vi "elab pictures 2d.vi"(8 "error in":errorcluster, 11 "path file in":path) -> (0 "error out":errorcluster)   [LabVIEW 2023]
uses:
  listbox/Selection Global Method.ctl
  <vilib>/Utility/file.llb/Read Delimited Spreadsheet (I64).vi
  queue/Front Panel Message Queue.lvlib
panel:
  in  "generate":bool
  in  "reset":bool
  out "all rows 2":i32[][][](array[numeric])
  out "all rows":i32[][][](array[numeric])
  in  "List Selected":T1(array[cluster])
  out "List Selected v":string[](array[string])
  out "List File":i32(listbox)
  in  "load":bool
  in  "Stop":bool
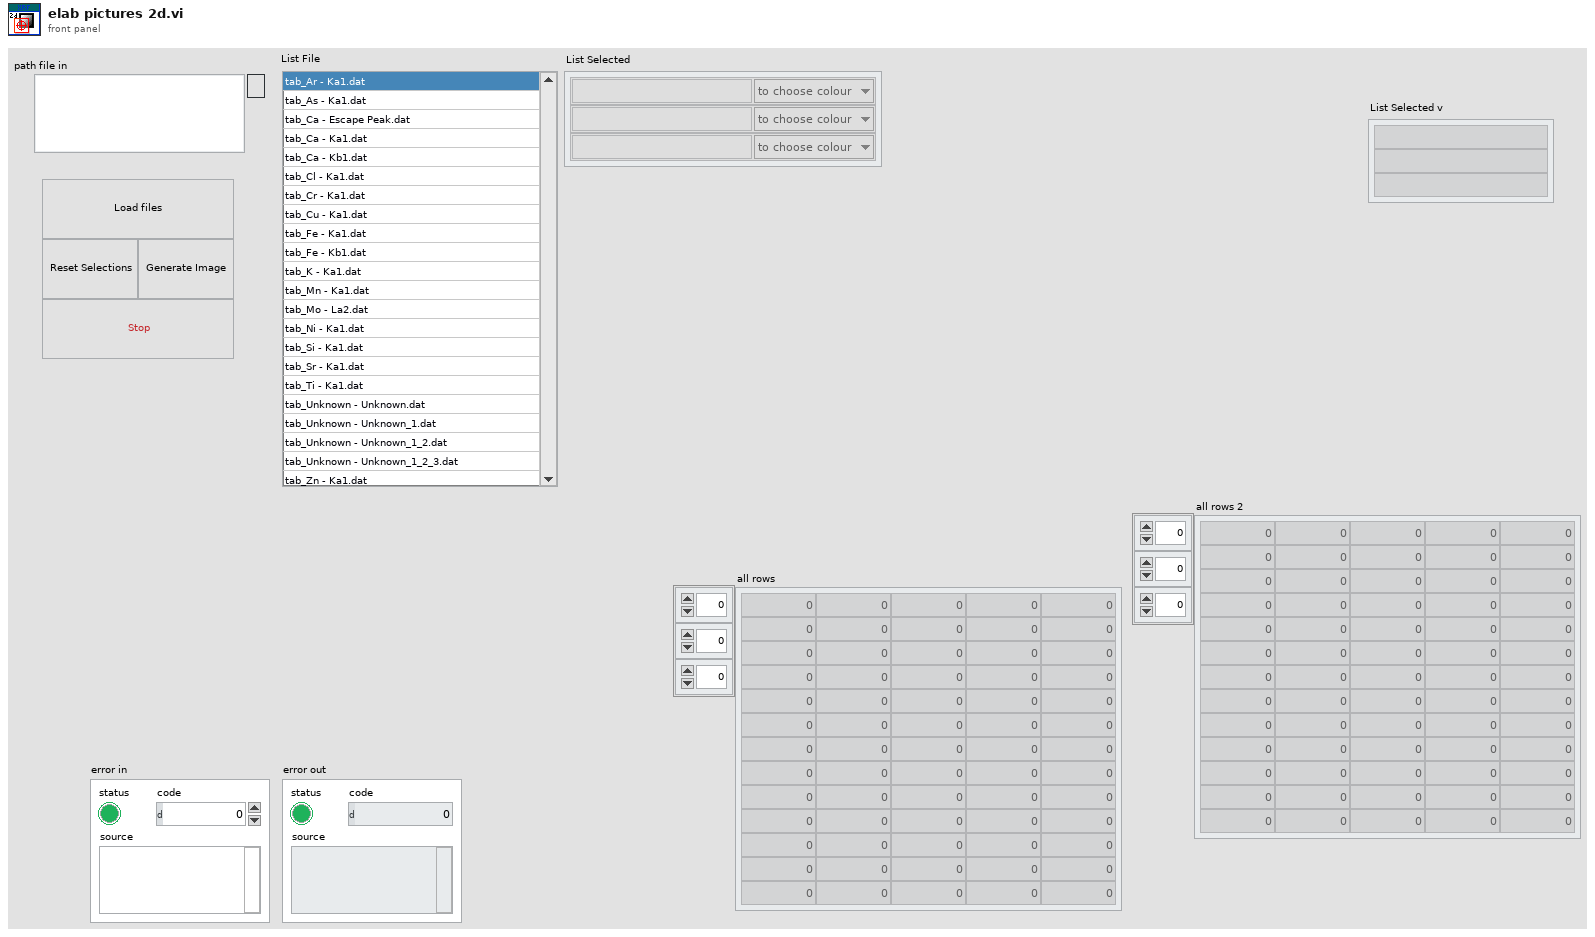
[diagram p1: front panel]
types:
  T1 = cluster{"Table":string, "color":enum16{"to choose colour", "red", "green", "blue"}}[]
  T2 = typedef "Front Panel Message Queue.lvlib/2d3d Message Queues.ctl" = cluster{"Main":refnum<queue>, "2d":refnum<queue>, "3d":refnum<queue>}
  T3 = typedef "Selection Global Method.ctl" = enum16{"Read Selection", "Force Selection", "Mouse Down Event", "Select All", "Select None", "Invert Selection", "Read Selection and Tags"}
  T4 = cluster{"Red name":string, "Green name":string, "Blu name":string}
  T5 = cluster{"Table":string, "color":enum16{"to choose colour", "red", "green", "blue"}}
  T6 = enum16{"to choose colour", "red", "green", "blue"}
  T7 = typedef "LVPoint32TypeDef.ctl" = cluster{"Horizontal":i32, "Vertical":i32}
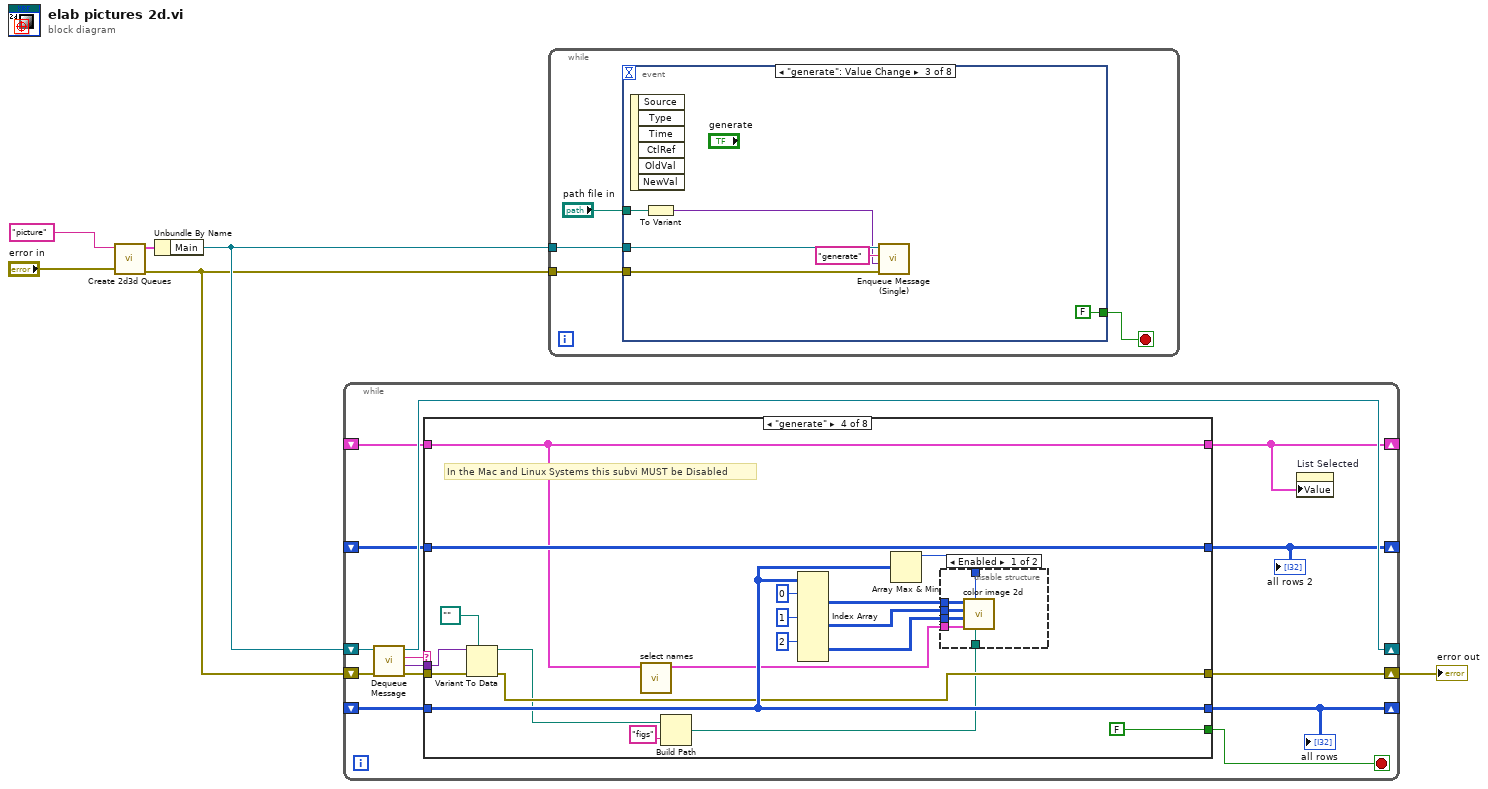
[diagram p0: block diagram]
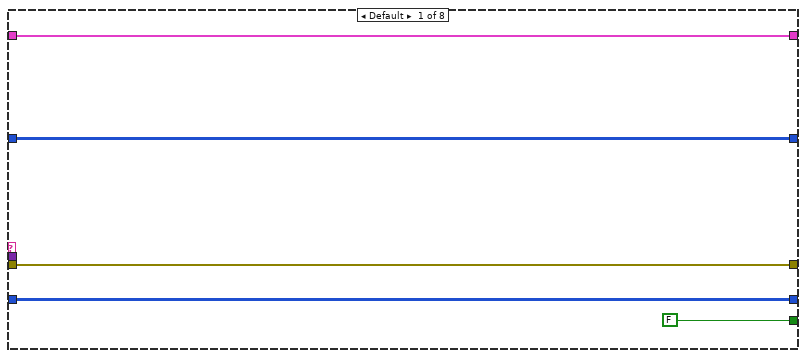
[diagram p2: hidden frame]
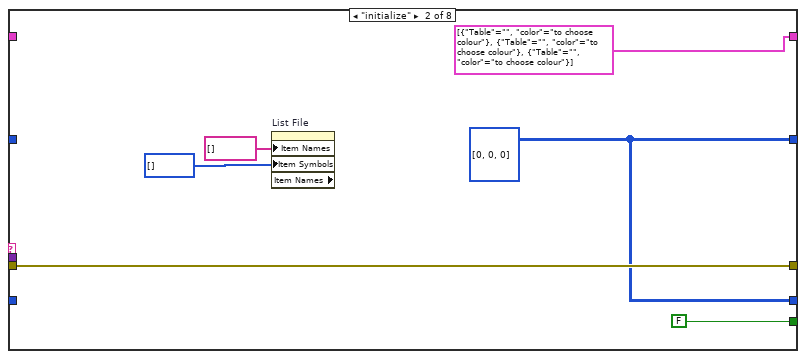
[diagram p3: hidden frame]
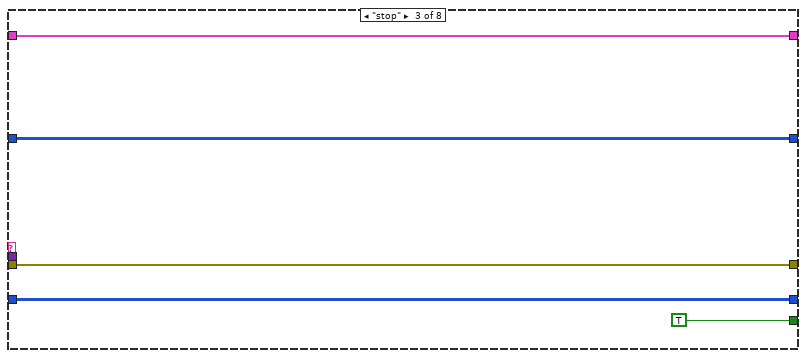
[diagram p4: hidden frame]
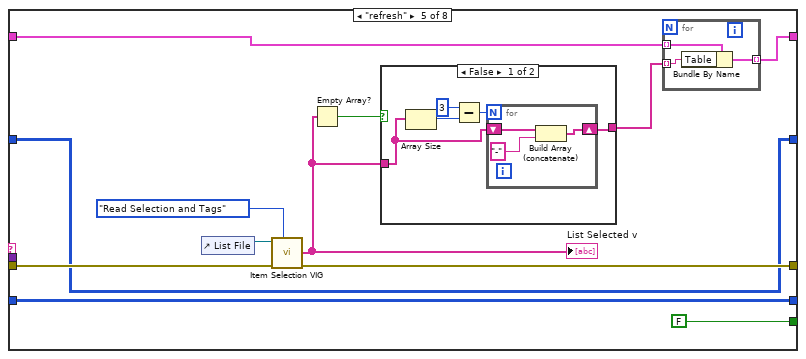
[diagram p6: hidden frame]
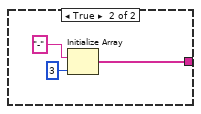
[diagram p7: hidden frame]
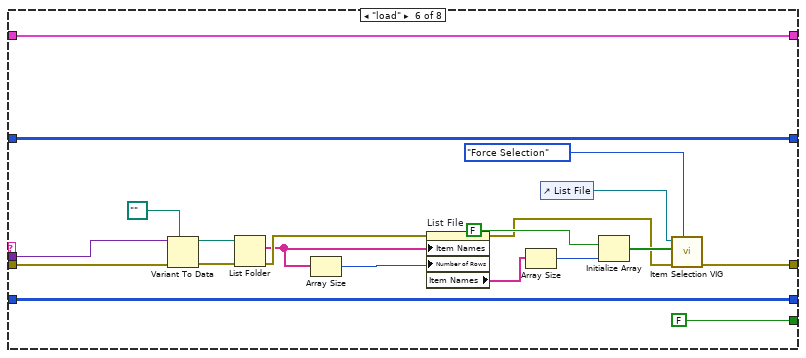
[diagram p8: hidden frame]
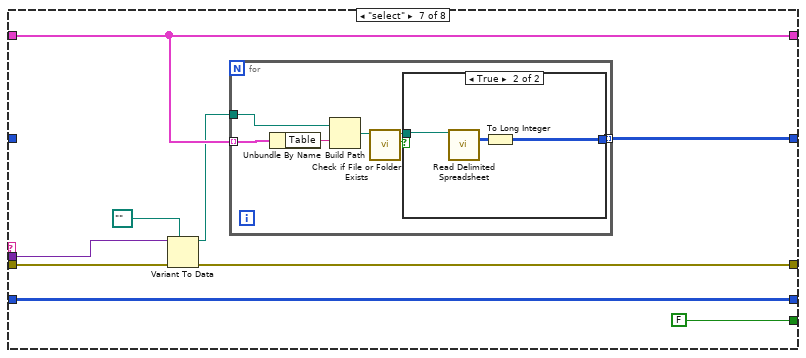
[diagram p9: hidden frame]
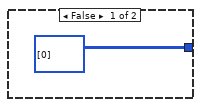
[diagram p10: hidden frame]
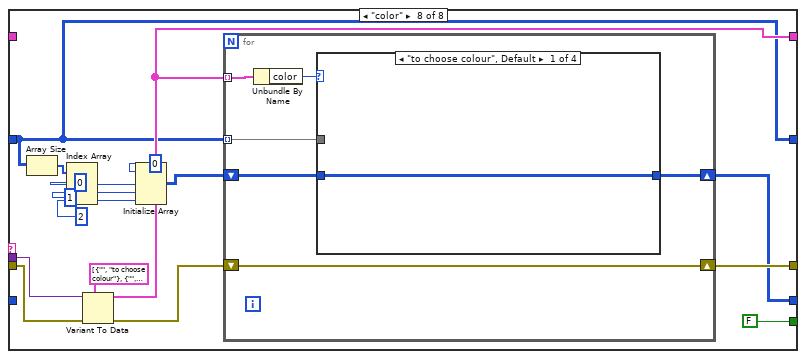
[diagram p11: hidden frame]
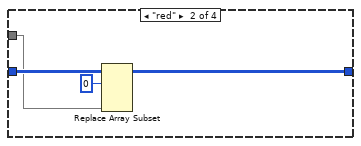
[diagram p12: hidden frame]
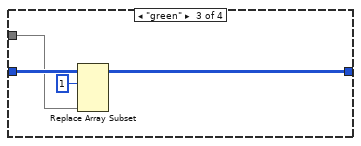
[diagram p13: hidden frame]
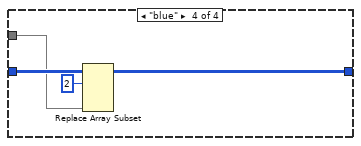
[diagram p14: hidden frame]
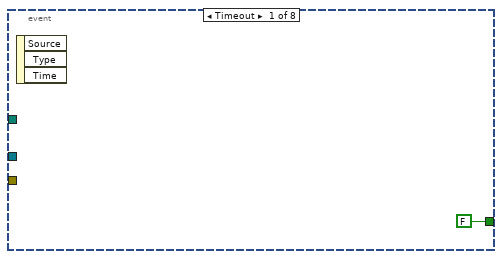
[diagram p15: hidden frame]
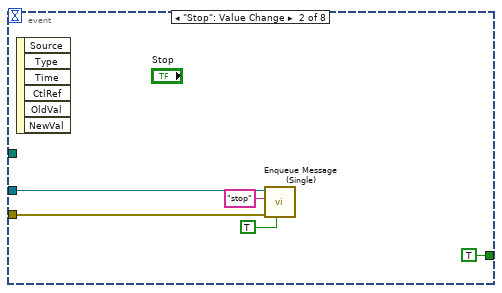
[diagram p16: hidden frame]
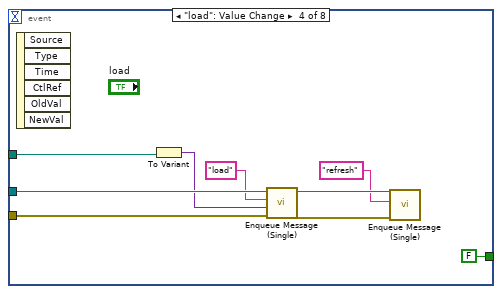
[diagram p17: hidden frame]
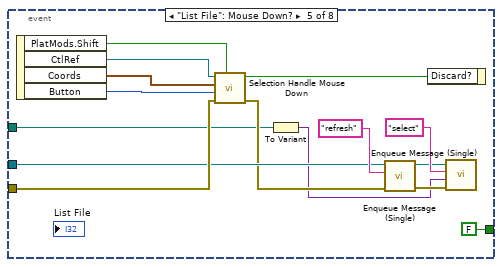
[diagram p18: hidden frame]
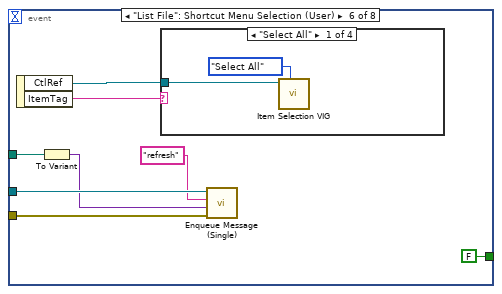
[diagram p19: hidden frame]
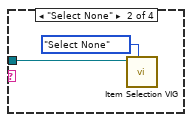
[diagram p20: hidden frame]
diagram:
  n1 = call "Create 2d3d Queues.vi"("error in (no error)"="error in", "name"="picture") -> ("error out"=w2:errorcluster, "Message Queues"=w4:T2)  [unwired: 8 in]
  n2 = Unbundle By Name(w4) -> ("Main"=w3:refnum<queue>)
  n3 = while {
    shift-right: [w13] -> _
    shift-left: w3 -> [w20]
    shift-right: [w17] -> w1
    shift-left: w2 -> [w19]
    shift-right: [w11] -> _
    shift-left: _ -> [w12]
    shift-right: [w10] -> _
    shift-left: _ -> [w9]
    shift-right: [w8] -> _
    shift-left: _ -> [w7]
    stop <- w15 stop-if-true
    n4 = call "Dequeue Message.vi"("error in (no error)"=w19, "Message Queue"=w20) -> ("error out"=w16:errorcluster, "Message Data"=w14:variant, "Message"=w18:string, "dup Message Queue"=w13:refnum<queue>)  [unwired: 5 in, 1 out]
    n5 = case shown="\"generate\"" w18 {
      tunnel: [w25 w28 w32 w40 w70 w91 w112 w144] -> w17
      tunnel: w16 -> [w25 w28 w32 w43 w69 w106 w115 w142]
      tunnel: [FALSE FALSE TRUE FALSE FALSE FALSE FALSE FALSE] -> w15
      tunnel: w14 -> [_ _ _ w42 _ w104 w113 w140]
      tunnel: w12 -> [w23 _ w33 w45 w68 w90 w111 _]
      tunnel: [w23 T1 [{"Table"="", "color"=enum."to choose colour"}, {"Table"="", "color"=enum."to choose colour"}, {"Table"="", "color"=enum."to choose colour"}] ("List Selected") w33 w45 w67 w90 w111 w138] -> w11
      tunnel: [w22 w26 w35 w54 w63 w89 w109 w136] -> w10
      tunnel: w9 -> [w22 _ w35 w54 w63 w89 _ w136]
      tunnel: [w21 w26 w34 w46 w62 w88 w108 w143] -> w8
      tunnel: w7 -> [w21 _ w34 w46 w62 w88 w108 _]
      frame Default {
      }
      frame "initialize" {
        w26 = i32[][][] [[[0]], [[0]], [[0]]] ("all rows")
        n6 = property on="List File" class="LstBox (strict)" props=["Item Names", "Item Symbols", "Item Names"]("Item Names"=string[] [], "Item Symbols"=i32[] []) -> ()  [unwired: 2 in, 3 out]
      }
      frame "stop" {
      }
      frame "generate" {
        # "In the Mac and Linux Systems this subvi MUST be Disabled"
        n7 = Variant To Data(error in=w43, type=path "", Variant=w42) -> (data=w39:path, error out=w40:errorcluster)
        n8 = call "select names.vi"("List Selected"=w45) -> ("Names"=w44:T4)  [unwired: 10 in]
        n9 = Build Path(base path=w39, name or relative path="figs") -> (appended path=w37:path)
        n10 = Index Array(array=w46, index (dim 0) #1=0 ("index (page)"), index (dim 0) #2=1 ("index (page)"), index (dim 0) #3=2 ("index (page)")) -> (element #1=w50:i32[][], element #2=w51:i32[][], element #3=w52:i32[][])  [unwired: 6 in]
        n11 = Array Max & Min(array=w46) -> (max value=w53:i32)  [unwired: 3 out]
        n12 = disable-structure "Diagram Disable Structure" shown="Enabled" {
          disable-tunnel: w53 -> [w61 _]
          disable-tunnel: w52 -> [w60 _]
          disable-tunnel: w51 -> [w59 _]
          disable-tunnel: w50 -> [w58 _]
          disable-tunnel: w44 -> [w57 _]
          disable-tunnel: w37 -> [w56 _]
          frame Enabled {
            n13 = call "color image 2d.vi"("path to JPEG file"=w56, "Max"=w61, "Names"=w57, "ROI-Blue"=w60, "ROI-Green"=w59, "ROI-Red"=w58) -> ()  [unwired: 6 in]
          }
          frame Disabled {
          }
        }
      }
      frame "refresh" {
        n14 = control-ref of="List File"() -> (w71:refnum<vi>)
        n15 = call "Item Selection VIG.vi"("Method (Read Selection)"=Selection_Global_Method."Read Selection and Tags", "error in (no error)"=w69, "Listbox or Tree"=w71) -> ("error out"=w70:errorcluster, "Tags"=w64:string[])  [unwired: 6 in, 1 out]
        "List Selected v" <- w64
        n16 = Empty Array?(array=w64) -> (empty?=w66:bool)
        n17 = case shown="False" w66 {
          tunnel: [w75 w82] -> w65
          tunnel: w64 -> [w74 _]
          frame False {
            n18 = Array Size(array=w74) -> (size(s)=w77:i32)
            n19 = Subtract(x=3, y=w77) -> (x-y=w78:i32)
            n20 = for {
              N: w78 -> [_]
              shift-right: [w79] -> w75
              shift-left: w74 -> [w81]
              n21 = Build Array (concatenate)(w81, "-") -> (w79:string[])
            }
          }
          frame True {
            n22 = Initialize Array("-", 3 ("dimension size")) -> (w82:string[])
          }
        }
        n23 = for {
          tunnel: w65 -> [w86] mode=indexing
          tunnel: w68 -> [w87] mode=indexing
          tunnel: [w85] -> w67 mode=indexing
          n24 = Bundle By Name(cluster=w87, "Table"=w86) -> (w85:T5)
        }
      }
      frame "load" {
        n25 = Variant To Data(error in=w106, type=path "", Variant=w104) -> (data=w102:path, error out=w103:errorcluster)
        n26 = List Folder(path=w102, error in=w103) -> (filenames=w99:string[], error out=w101:errorcluster)  [unwired: 2 in, 2 out]
        n27 = Array Size(array=w99) -> (size(s)=w100:i32)
        n28 = property on="List File" class="LstBox (strict)"(error in=w101, "Item Names"=w99, "Number of Rows"=w100) -> (error out=w92:errorcluster, "Item Names"=w93:string[])  [unwired: 1 in, 1 out]
        n29 = Array Size(array=w93) -> (size(s)=w98:i32)
        n30 = control-ref of="List File"() -> (w97:refnum<vi>)
        n31 = Initialize Array(FALSE, w98) -> (w96:bool[])
        n32 = call "Item Selection VIG.vi"("Method (Read Selection)"=Selection_Global_Method."Force Selection", "error in (no error)"=w92, "Selection"=w96, "Listbox or Tree"=w97) -> ("error out"=w91:errorcluster)  [unwired: 5 in, 2 out]
      }
      frame "select" {
        n33 = Variant To Data(error in=w115, type=path "", Variant=w113) -> (data=w110:path, error out=w112:errorcluster)
        n34 = for {
          tunnel: w111 -> [w123] mode=indexing
          tunnel: w110 -> [w121]
          tunnel: [w117] -> w109 mode=indexing
          n35 = Unbundle By Name(w123) -> ("Table"=w122:string)
          n36 = Build Path(base path=w121, name or relative path=w122) -> (appended path=w120:path)
          n37 = call <vilib>:"Check if File or Folder Exists.vi"("path"=w120) -> ("file or folder exists?"=w119:bool, "dup path"=w118:path)  [unwired: 8 in, 1 out]
          n38 = case shown="True" w119 {
            tunnel: w118 -> [_ w127]
            tunnel: [i32[][] [[0]] ("all rows") w125] -> w117
            frame False {
            }
            frame True {
              n39 = call-poly <vilib>:"Read Delimited Spreadsheet.vi"("file path (dialog if empty)"=w127) -> ("all rows"=w126:i64[][])  [unwired: 9 in, 5 out]
              n40 = To Long Integer(number=w126) -> (32bit integer=w125:i32[][])
            }
          }
        }
      }
      frame "color" {
        n41 = Array Size(array=w136) -> (size(s)=w135:i32[])
        n42 = Index Array(array=w135, index #1=0 ("index"), index #2=1 ("index"), index #3=2 ("index")) -> (element #1=w131:i32, element #2=w130:i32, element #3=w129:i32)
        n43 = Variant To Data(error in=w142, type=T1 [{"Table"="", "color"=enum."to choose colour"}, {"Table"="", "color"=enum."to choose colour"}, {"Table"="", "color"=enum."to choose colour"}] ("List Selected"), Variant=w140) -> (data=w138:T1, error out=w141:errorcluster)
        n44 = Initialize Array(0, w131, w130, w129) -> (w128:i32[][][])
        n45 = for {
          tunnel: w138 -> [w150] mode=indexing
          tunnel: w136 -> [w148] mode=indexing
          shift-right: [w151] -> w144
          shift-left: w141 -> [w151]
          shift-right: [w146] -> w143
          shift-left: w128 -> [w147]
          n46 = Unbundle By Name(w150) -> ("color"=w149:T6)
          n47 = case shown="\"to choose colour\", Default" w149 {
            tunnel: w148 -> [_ w154 w158 w162]
            tunnel: w147 -> [w152 w156 w159 w163]
            tunnel: [w152 w153 w157 w161] -> w146
            frame "to choose colour", Default {
            }
            frame "red" {
              n48 = Replace Array Subset(array=w156, new element=w154, index (dim 0)=0 ("index (page)")) -> (w153:i32[][][])  [unwired: 2 in]
            }
            frame "green" {
              n49 = Replace Array Subset(array=w159, new element=w158, index (dim 0)=1 ("index (page)")) -> (w157:i32[][][])  [unwired: 2 in]
            }
            frame "blue" {
              n50 = Replace Array Subset(array=w163, new element=w162, index (dim 0)=2 ("index (page)")) -> (w161:i32[][][])  [unwired: 2 in]
            }
          }
        }
      }
    }
    "all rows" <- w8
    "all rows 2" <- w10
    n51 = property on="List Selected" class="Arr (strict)"("Value"=w11) -> ()  [unwired: 2 in, 2 out]
  }
  "error out" <- w1
  n52 = while {
    tunnel: w3 -> [w168]
    tunnel: w2 -> [w167]
    stop <- w166 stop-if-true
    n53 = event shown="[2] \"generate\": Value Change" {
      selector: _ -> [_ _ _ _ _ _ _ _]
      dyn-events: _ -> [_ _ _ _ _ _ _ _]
      timeout: _ -> [_ _ _ _ _ _ _ _]
      tunnel: w168 -> [_ w173 w179 w188 w196 w211 w226 w232]
      tunnel: w167 -> [_ w172 w178 w187 w198 w210 w225 w233]
      tunnel: [FALSE TRUE FALSE FALSE FALSE FALSE FALSE FALSE] -> w166
      tunnel: "path file in" -> [_ _ w176 w184 w194 w208 w223 _]
      event Timeout {
        n54 = event-data() -> ()  [unwired: 1 in, 3 out]
      }
      event "Stop": Value Change {
        n55 = event-data() -> ()  [unwired: 1 in, 6 out]
        n56 = call "Enqueue Message (Single).vi"("Priority Message? (F)"=TRUE, "error in (no error)"=w172, "Message"="stop", "Message Queue"=w173) -> ()  [unwired: 6 in, 2 out]
      }
      event "generate": Value Change {
        n57 = event-data() -> ()  [unwired: 1 in, 6 out]
        n58 = To Variant(anything=w176) -> (Variant=w175:variant)
        n59 = call "Enqueue Message (Single).vi"("error in (no error)"=w178, "Message Data"=w175, "Message"="generate", "Message Queue"=w179) -> ()  [unwired: 6 in, 2 out]
      }
      event "load": Value Change {
        n60 = event-data() -> ()  [unwired: 1 in, 6 out]
        n61 = To Variant(anything=w184) -> (Variant=w185:variant)
        n62 = call "Enqueue Message (Single).vi"("error in (no error)"=w187, "Message Data"=w185, "Message"="load", "Message Queue"=w188) -> ("error out"=w183:errorcluster, "dup Message Queue"=w182:refnum<queue>)  [unwired: 6 in]
        n63 = call "Enqueue Message (Single).vi"("error in (no error)"=w183, "Message"="refresh", "Message Queue"=w182) -> ()  [unwired: 7 in, 2 out]
      }
      event "List File": Mouse Down? {
        n64 = event-data() -> ("PlatMods.Shift"=w200:bool, "CtlRef"=w201:refnum<vi>, "Coords"=w202:T7, "Button"=w203:u16)  [unwired: 1 in]
        n65 = call "Selection Handle Mouse Down.vi"("Shift?"=w200, "error in (no error)"=w198, "Mouse Button"=w203, "Mouse Coords"=w202, "Listbox or Tree"=w201) -> ("error out"=w195:errorcluster, "Discard?"=w199:bool)  [unwired: 5 in]
        n66 = To Variant(anything=w194) -> (Variant=w190:variant)
        n67 = call "Enqueue Message (Single).vi"("error in (no error)"=w195, "Message"="refresh", "Message Queue"=w196) -> ("error out"=w191:errorcluster, "dup Message Queue"=w192:refnum<queue>)  [unwired: 7 in]
        n68 = event-data("Discard?"=w199) -> ()  [unwired: 1 in, 1 out]
        n69 = call "Enqueue Message (Single).vi"("error in (no error)"=w191, "Message Data"=w190, "Message"="select", "Message Queue"=w192) -> ()  [unwired: 6 in, 2 out]
      }
      event "List File": Shortcut Menu Selection (User) {
        n70 = event-data() -> ("CtlRef"=w205:refnum<vi>, "ItemTag"=w206:string)  [unwired: 1 in]
        n71 = To Variant(anything=w208) -> (Variant=w207:variant)
        n72 = case shown="\"Select All\"" w206 {
          tunnel: w205 -> [w214 w216 w218 _]
          frame "Select All" {
            n73 = call "Item Selection VIG.vi"("Method (Read Selection)"=Selection_Global_Method."Select All", "Listbox or Tree"=w214) -> ()  [unwired: 7 in, 3 out]
          }
          frame "Select None" {
            n74 = call "Item Selection VIG.vi"("Method (Read Selection)"=Selection_Global_Method."Select None", "Listbox or Tree"=w216) -> ()  [unwired: 7 in, 3 out]
          }
          frame "Invert Selection" {
            n75 = call "Item Selection VIG.vi"("Method (Read Selection)"=Selection_Global_Method."Invert Selection", "Listbox or Tree"=w218) -> ()  [unwired: 7 in, 3 out]
          }
          frame Default {
          }
        }
        n76 = call "Enqueue Message (Single).vi"("error in (no error)"=w210, "Message Data"=w207, "Message"="refresh", "Message Queue"=w211) -> ()  [unwired: 6 in, 2 out]
      }
      event "reset": Value Change {
        n77 = event-data() -> ()  [unwired: 1 in, 3 out]
        n78 = To Variant(anything=w223) -> (Variant=w222:variant)
        n79 = control-ref of="List File"() -> (w220:refnum<vi>)
        n80 = call "Enqueue Message (Single).vi"("error in (no error)"=w225, "Message Data"=w222, "Message"="refresh", "Message Queue"=w226) -> ("error out"=w219:errorcluster)  [unwired: 6 in, 1 out]
        n81 = call "Item Selection VIG.vi"("Method (Read Selection)"=Selection_Global_Method."Select None", "error in (no error)"=w219, "Listbox or Tree"=w220) -> ()  [unwired: 6 in, 3 out]
      }
      event "List Selected": Value Change {
        n82 = event-data() -> ("NewVal"=w229:T1)  [unwired: 1 in, 5 out]
        n83 = To Variant(anything=w229) -> (Variant=w228:variant)
        n84 = call "Enqueue Message (Single).vi"("error in (no error)"=w233, "Message Data"=w228, "Message"="color", "Message Queue"=w232) -> ()  [unwired: 6 in, 2 out]
      }
    }
  }
